vi "KT数据判定.vi"(7 "data in":u16[](array[numeric])) -> (8 "result":bool)   [LabVIEW 2016]
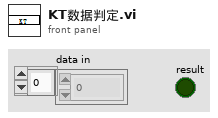
[diagram p1: front panel]
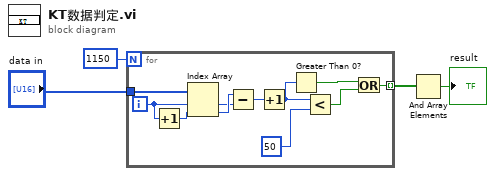
[diagram p0: block diagram]
diagram:
  n1 = for {
    N: 1150 -> [_]
    tunnel: "data in" -> [w15]
    tunnel: [w6] -> w3 mode=indexing
    i -> [w13]
    n2 = Increment(x=w13) -> (x+1=w14:i32)
    n3 = Index Array(array=w15, index #1=w13, index #2=w14) -> (element #1=w11:u16, element #2=w12:u16)
    n4 = Subtract(x=w12, y=w11) -> (x-y=w10:u16)
    n5 = Increment(x=w10) -> (x+1=w5:u16)
    n6 = Greater Than 0?(x=w5) -> (x > 0?=w8:bool)
    n7 = Less?(x=w5, y=u16 50) -> (x < y?=w7:bool)
    n8 = Or(x=w8, y=w7) -> (x .or. y?=w6:bool)
  }
  n9 = And Array Elements(Boolean array=w3) -> (logical AND=→"result":bool)
